vi "CalcCksum.vi"(1 "Byte Cnt":u16, 2 "Buffer":u8[](array[numeric])) -> (0 "CkSum":u16)   [LabVIEW 2016]
panel:
  out "Odd Bytes":u8
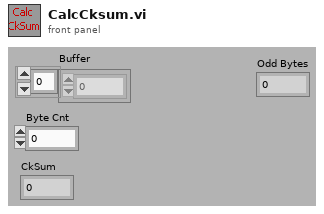
[diagram p1: front panel]
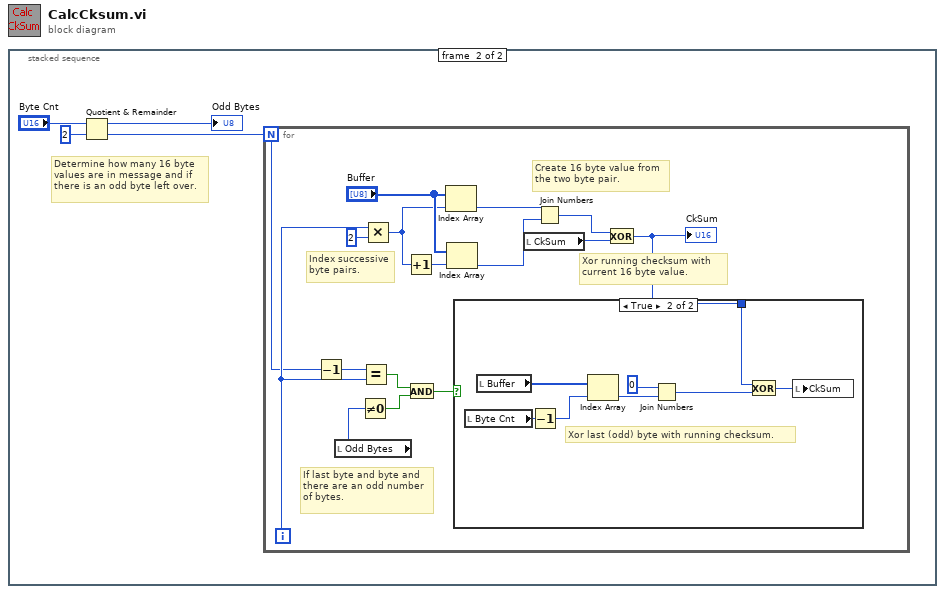
[diagram p0: block diagram]
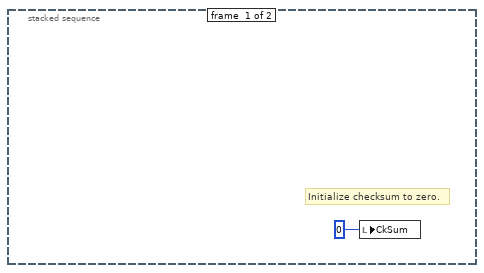
[diagram p2: hidden frame]
diagram:
  n1 = stacked-sequence {
    frame #0 {
      # "Initialize checksum to zero."
      n2 = local write "CkSum"(u16 0 ("CkSum")) -> ()
    }
    frame #1 {
      # "Determine how many 16 byte\nvalues are in message and if\nthere is an odd byte left over."
      n3 = Quotient & Remainder(x="Byte Cnt", y=u16 2) -> (x-y*floor(x/y)=→"Odd Bytes":u16, floor(x/y)=w2:u16)
      n4 = for {
        N: w2 -> [w8]
        i -> [w15]
        # "If last byte and byte and\nthere are an odd number\nof bytes."
        # "Index successive\nbyte pairs."
        # "Xor running checksum with\ncurrent 16 byte value."
        # "Create 16 byte value from\nthe two byte pair."
        n5 = Decrement(x=w8) -> (x-1=w9:i32)
        n6 = local read "Odd Bytes"() -> (w14:u8)
        n7 = Not Equal To 0?(x=w14) -> (x != 0?=w12:bool)
        n8 = Equal?(x=w9, y=w15) -> (x = y?=w13:bool)
        n9 = Multiply(x=w15, y=u16 2) -> (x*y=w6:i32)
        n10 = Increment(x=w6) -> (x+1=w7:i32)
        n11 = And(x=w13, y=w12) -> (x .and. y?=w11:bool)
        n12 = Index Array "Index Array"(array="Buffer", index=w6) -> (element=w19:u8)
        n13 = Index Array "Index Array"(array="Buffer", index=w7) -> (element=w18:u8)
        n14 = local read "CkSum"() -> (w16:u16)
        n15 = Join Numbers(hi=w19, lo=w18) -> ((hi.lo)=w17:u16)
        n16 = Exclusive Or(1:w16, 2:w17) -> (0:w10:u16)
        "CkSum" <- w10
        n17 = case shown="True" w11 {
          tunnel: w10 -> [_ w23]
          frame False {
          }
          frame True {
            # "Xor last (odd) byte with running checksum."
            n18 = local read "Byte Cnt"() -> (w28:u16)
            n19 = local read "Buffer"() -> (w29:u8[])
            n20 = Decrement(x=w28) -> (x-1=w27:u16)
            n21 = Index Array "Index Array"(array=w29, index=w27) -> (element=w25:u8)
            n22 = Join Numbers(hi=u8 0 ("lo"), lo=w25) -> ((hi.lo)=w26:u16)
            n23 = Exclusive Or(1:w26, 2:w23) -> (0:w22:u16)
            n24 = local write "CkSum"(w22) -> ()
          }
        }
      }
    }
  }
